vi "EmsAndLimitTest.vi"() -> ()   [LabVIEW 2020]
uses:
  <vilib>/CISH Robotics/L4VMX VMXpi/Type Def/VMX Channel Index.ctl
  <vilib>/CISH Robotics/L4VMX VMXpi/Digital Input/Digital Input.lvclass
  <vilib>/CISH Robotics/L4VMX VMXpi/L4VMX.lvlib
panel:
  in  "Stop Button":bool
  out "zAxisLimit":bool
  out "EMS":bool
  # "EMS:DI8\nzAxisLimit:DI9"
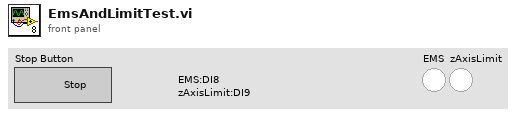
[diagram p1: front panel]
types:
  T1 = typedef "L4VMX.lvlib/VMX Channel Index.ctl" = enum16{"0", "1", "2", "3", "4", "5", "6", "7", "8", "9", "10", "11", "12", "13", "14", "15", "16", "17", "18", "19", "20", "21", "22", "23", "24", "25", "26", "27", "28", "29", "30", "31", "32", "33"}
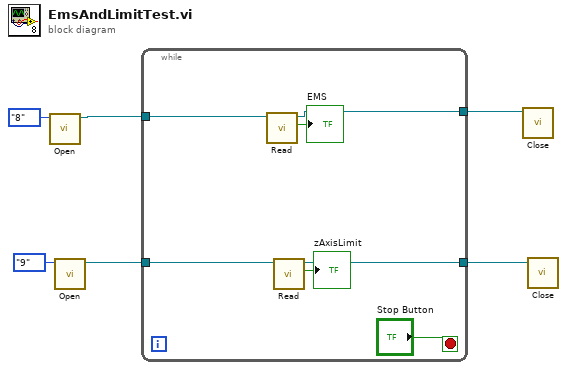
[diagram p0: block diagram]
diagram:
  n1 = call <vilib>:"Open.vi"("VMX Channel Index"=VMX_Channel_Index."8") -> ("Digital Input Object"=w6:refnum<class "Digital Input.lvclass">)  [unwired: 9 in, 1 out]
  n2 = call <vilib>:"Open.vi"("VMX Channel Index"=VMX_Channel_Index."9") -> ("Digital Input Object"=w4:refnum<class "Digital Input.lvclass">)  [unwired: 9 in, 1 out]
  n3 = while {
    tunnel: w6 -> [w13]
    tunnel: [w12] -> w5
    tunnel: w4 -> [w11]
    tunnel: [w10] -> w3
    stop <- "Stop Button" stop-if-true
    n4 = call <vilib>:"Read.vi"("Digital Input Object"=w13) -> ("Value"=→"EMS":bool, "Digital Input Object"=w12:refnum<class "Digital Input.lvclass">)  [unwired: 8 in, 1 out]
    n5 = call <vilib>:"Read.vi"("Digital Input Object"=w11) -> ("Value"=→"zAxisLimit":bool, "Digital Input Object"=w10:refnum<class "Digital Input.lvclass">)  [unwired: 8 in, 1 out]
  }
  n6 = call <vilib>:"Close.vi"("Digital Input Object"=w5) -> ()  [unwired: 10 in, 1 out]
  n7 = call <vilib>:"Close.vi"("Digital Input Object"=w3) -> ()  [unwired: 10 in, 1 out]
